vi "Write Default Funnel Cluster.vi"(8 "error in (no error)":errorcluster, 10 "Default Funnel":T1, 11 "Funnel Settings in":refnum<class "Funnel Settings.lvclass">) -> (0 "error out":errorcluster, 3 "Funnel Settings out":refnum<class "Funnel Settings.lvclass">)   [LabVIEW 2019, in "Funnel Settings.lvclass"]
uses:
  Funnel Settings.lvclass
  Typedefs/Default Funnel Cluster.ctl
  Funnel Settings.lvclass/Funnel Settings.ctl
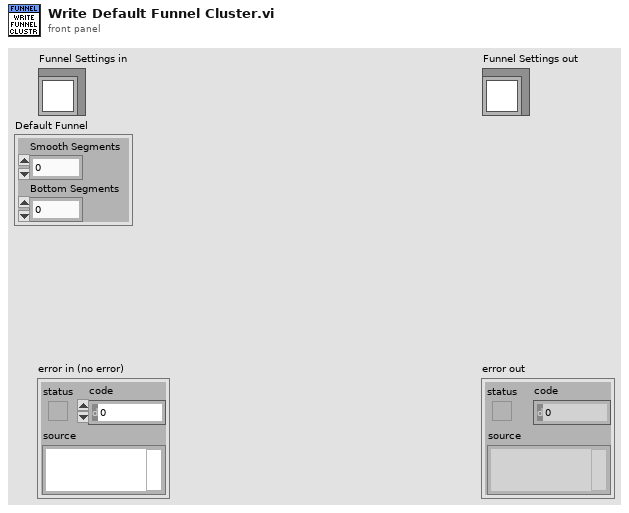
[diagram p1: front panel]
types:
  T1 = typedef "Funnel Settings.lvclass/Default Funnel Cluster.ctl" = cluster{"Smooth Segments":dbl, "Bottom Segments":dbl}
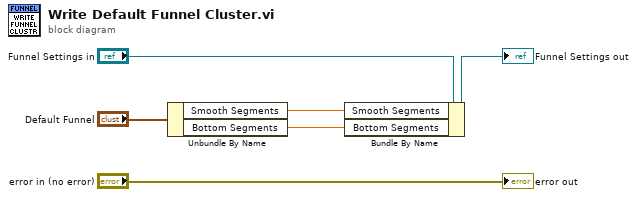
[diagram p0: block diagram]
diagram:
  n1 = Unbundle By Name("Default Funnel") -> ("Smooth Segments"=w3:dbl, "Bottom Segments"=w2:dbl)
  n2 = Bundle By Name(cluster="Funnel Settings in", "Smooth Segments"=w3, "Bottom Segments"=w2) -> (→"Funnel Settings out":refnum<class "Funnel Settings.lvclass">)
  "error out" <- "error in (no error)"
